vi "Cleanup.vi"(8 "error in (no error)":errorcluster, 11 "User DB in":refnum<class "User DB.lvclass">) -> (0 "error out":errorcluster)   [LabVIEW 2020, in "Summer of LabVIEW.lvlib" / "User DB.lvclass"]
uses:
  User DB.lvclass
  User DB.lvclass/User DB.ctl
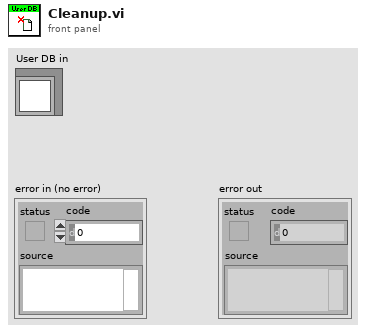
[diagram p1: front panel]
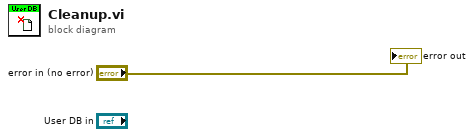
[diagram p0: block diagram]
diagram:
  "error out" <- "error in (no error)"
